vi "Find Goal Angle Difference.vi"(6 "Goal Display 2":T1(plugin-control), 7 "Offset":dbl, 10 "Normalized Rect":T2, 11 "Camera Type":T3) -> (3 "Angle Diff":dbl)   [LabVIEW 2015]
uses:
  Camera Types.ctl
panel:
  out "Distance (d)":dbl
  out "Center Offset (z)":dbl
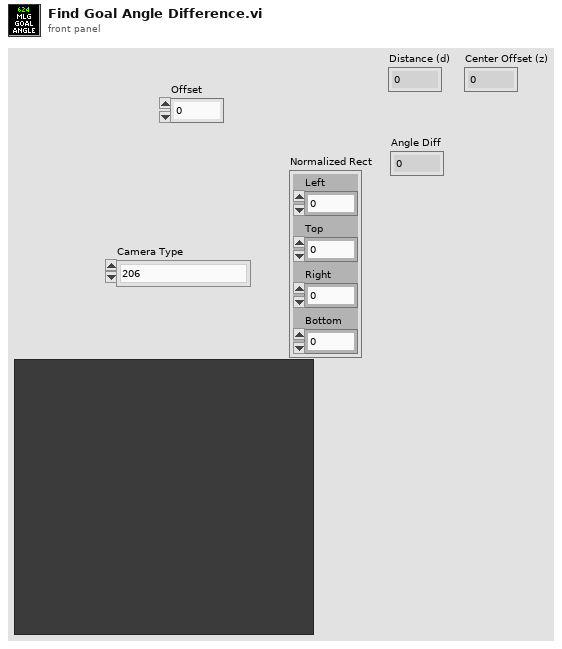
[diagram p1: front panel]
types:
  T1 = typedef "IMAQ Image.ctl" = refnum<image>
  T2 = cluster{"Left":dbl, "Top":dbl, "Right":dbl, "Bottom":dbl}
  T3 = typedef "Camera Types.ctl" = enum16{"206", "1011", "1013", "MS HD3000 square", "MS HD3000 640x480"}
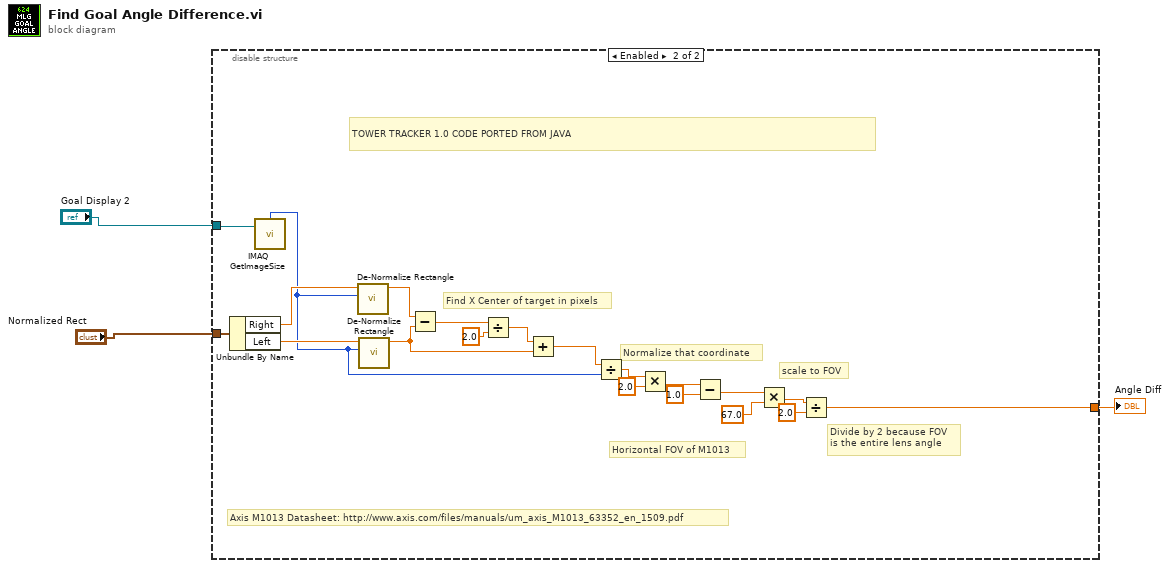
[diagram p0: block diagram]
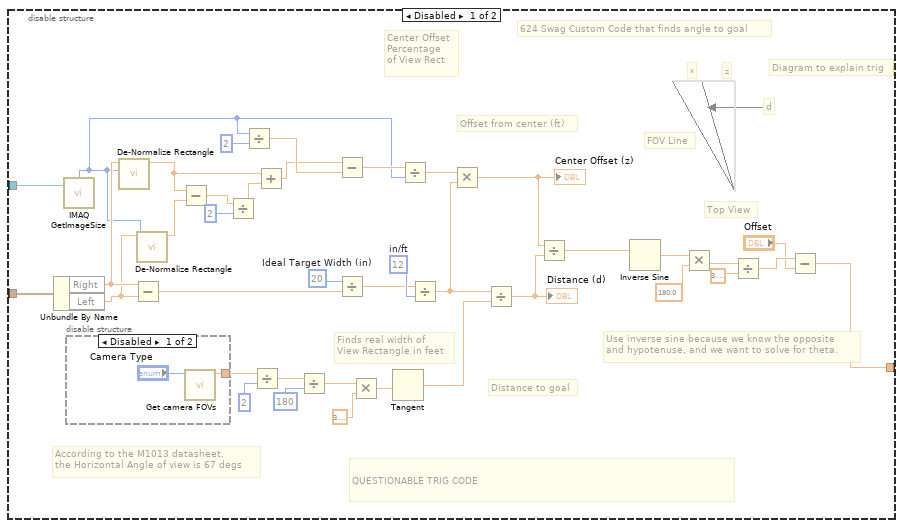
[diagram p2: hidden frame]
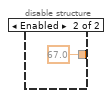
[diagram p3: hidden frame]
diagram:
  n1 = disable-structure shown="Enabled" {
    disable-tunnel: "Normalized Rect" -> [w6 w64]
    disable-tunnel: "Goal Display 2" -> [w5 w62]
    disable-tunnel: [w4 w45] -> w1
    frame Disabled {
      w33 = 20  # Ideal Target Width (in)
      w36 = 12  # in/ft
      # "QUESTIONABLE TRIG CODE"
      # "Use inverse sine because we know the opposite\nand hypotenuse, and we want to solve for theta."
      # "Diagram to explain trig"
      # "Top View"
      # "According to the M1013 datasheet,\nthe Horizontal Angle of view is 67 degs"
      # "FOV Line"
      # "d"
      # "z"
      # "x"
      # "Center Offset\nPercentage \nof View Rect"
      # "Distance to goal"
      # "Offset from center (ft)"
      # "Finds real width of \nView Rectangle in feet"
      # "624 Swag Custom Code that finds angle to goal"
      n2 = Unbundle By Name(w6) -> ("Right"=w29:dbl, "Left"=w14:dbl)
      n3 = call "IMAQ GetImageSize"("Image"=w5) -> ("X Resolution"=w15:i32)  [unwired: 3 in, 2 out]
      n4 = disable-structure shown="Disabled" {
        disable-tunnel: [w43 67.0 ("FOV")] -> w34
        frame Disabled {
          n5 = call "Get camera FOVs.vi"("Camera Type"="Camera Type") -> ("FOV"=w43:dbl)  [unwired: 9 in, 1 out]
        }
        frame Enabled {
        }
      }
      n6 = call "De-Normalize Rectangle.vi"("X Resolution"=w15, "Right"=w29) -> ("Pixels"=w9:dbl)  [unwired: 9 in]
      n7 = Subtract(x=w29, y=w14) -> (x-y=w30:dbl)
      n8 = call "De-Normalize Rectangle.vi"("X Resolution"=w15, "Right"=w14) -> ("Pixels"=w13:dbl)  [unwired: 9 in]
      n9 = Subtract(x=w9, y=w13) -> (x-y=w11:dbl)
      n10 = Divide(x=w11, y=2) -> (x/y=w10:dbl)
      n11 = Divide(x=w15, y=2) -> (x/y=w17:dbl)
      n12 = Divide(x=w34, y=2) -> (x/y=w39:dbl)
      n13 = Add(x=w9, y=w10) -> (x+y=w8:dbl)
      n14 = Divide(x=w39, y=180) -> (x/y=w38:dbl)
      n15 = Subtract(x=w8, y=w17) -> (x-y=w16:dbl)
      n16 = Divide(x=w33, y=w30) -> (x/y=w35:dbl)
      n17 = Multiply(x=w38, y=3.141592653589793) -> (x*y=w40:dbl)
      n18 = Tangent(1:w40) -> (0:w32:dbl)
      n19 = Divide(x=w16, y=w15) -> (x/y=w28:dbl)
      n20 = Divide(x=w35, y=w36) -> (x/y=w27:dbl)
      n21 = Multiply(x=w28, y=w27) -> (x*y=w26:dbl)
      "Center Offset (z)" <- w26
      n22 = Divide(x=w27, y=w32) -> (x/y=w25:dbl)
      "Distance (d)" <- w25
      n23 = Divide(x=w26, y=w25) -> (x/y=w24:dbl)
      n24 = Inverse Sine(1:w24) -> (0:w20:dbl)
      n25 = Multiply(x=w20, y=180.0) -> (x*y=w22:dbl)
      n26 = Divide(x=w22, y=3.141592653589793) -> (x/y=w19:dbl)
      n27 = Subtract(x=w19, y="Offset") -> (x-y=w4:dbl)
    }
    frame Enabled {
      # "Axis M1013 Datasheet: http://www.axis.com/files/manuals/um_axis_M1013_63352_en_1509.pdf"
      # "Divide by 2 because FOV\nis the entire lens angle"
      # "Horizontal FOV of M1013"
      # "scale to FOV"
      # "Normalize that coordinate"
      # "Find X Center of target in pixels"
      # "TOWER TRACKER 1.0 CODE PORTED FROM JAVA"
      n28 = Unbundle By Name(w64) -> ("Right"=w61:dbl, "Left"=w63:dbl)
      n29 = call "IMAQ GetImageSize"("Image"=w62) -> ("X Resolution"=w54:i32)  [unwired: 3 in, 2 out]
      n30 = call "De-Normalize Rectangle.vi"("X Resolution"=w54, "Right"=w61) -> ("Pixels"=w60:dbl)  [unwired: 9 in]
      n31 = call "De-Normalize Rectangle.vi"("X Resolution"=w54, "Right"=w63) -> ("Pixels"=w56:dbl)  [unwired: 9 in]
      n32 = Subtract(x=w60, y=w56) -> (x-y=w59:dbl)
      n33 = Divide(x=w59, y=2.0) -> (x/y=w57:dbl)
      n34 = Add(x=w57, y=w56) -> (x+y=w55:dbl)
      n35 = Divide(x=w55, y=w54) -> (x/y=w53:dbl)
      n36 = Multiply(x=w53, y=2.0) -> (x*y=w51:dbl)
      n37 = Subtract(x=w51, y=1.0) -> (x-y=w49:dbl)
      n38 = Multiply(x=w49, y=67.0) -> (x*y=w47:dbl)
      n39 = Divide(x=w47, y=2.0) -> (x/y=w45:dbl)
    }
  }
  "Angle Diff" <- w1
